vi "Shutdown.vi"(8 "error in (no error)":errorcluster, 11 "Stage_MadCityLab in":refnum<class "Stage_MadCityLab.lvclass">) -> (0 "error out":errorcluster, 3 "Stage_MadCityLab out":refnum<class "Stage_MadCityLab.lvclass">)   [LabVIEW 2020, in "Stage_MadCityLab.lvlib" / "Stage_MadCityLab.lvclass"]
uses:
  Stage_MadCityLab.lvclass
  Stage_MadCityLab.lvclass/Stage_MadCityLab.ctl
  HAL Layer/Component/Stage/Stage/Stage.lvclass
  Dependency/Madlib.dll
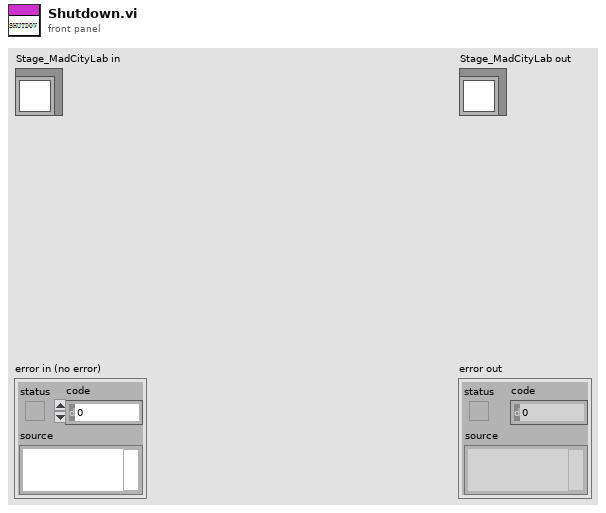
[diagram p1: front panel]
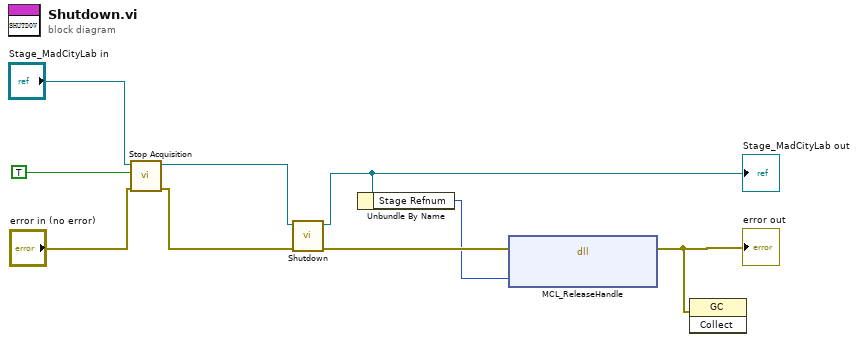
[diagram p0: block diagram]
diagram:
  n1 = call-dynamic "Stop Acquisition.vi"("Stage in"="Stage_MadCityLab in", "Stop"=TRUE, "error in (no error)"="error in (no error)") -> ("Stage out"=w8:refnum<class "Stage_MadCityLab.lvclass">, "error out"=w6:errorcluster)  [unwired: 6 in]
  n2 = call-parent "Shutdown.vi"("error in (no error)"=w6, "Device in"=w8) -> ("error out"=w4:errorcluster, "Device out"=w3:refnum<class "Stage_MadCityLab.lvclass">)  [unwired: 8 in]
  "Stage_MadCityLab out" <- w3
  n3 = Unbundle By Name(w3) -> ("Stage Refnum"=w2:i32)
  n4 = dll-call lib="D:/Daguan/Development/MMicroscopyAF/Model/Real Hardware/Stage_MadCityLab/Stage_MadCityLab/Dependency/Madlib.dll" fn="MCL_ReleaseHandle"(error in=w4, "handle"=w2) -> (error out=w1:errorcluster)  [unwired: 3 in, 2 out]
  "error out" <- w1
  n5 = invoke class="GC" method="Collect"(error in=w1) -> ()  [unwired: 2 in, 3 out]
